vi "DisplayCurrentValues.vi"(8 "error in (no error)":errorcluster, 11 "Tare Currents?":bool) -> (0 "error out":errorcluster, 1 "PDP Energy (J)":dbl, 2 "PDP Current (A)":dbl[](array[numeric]), 3 "Sum of Current":dbl, 4 "PDP Power (W)":dbl)   [LabVIEW 2016]
panel:
  in  "Reset Energy?":bool
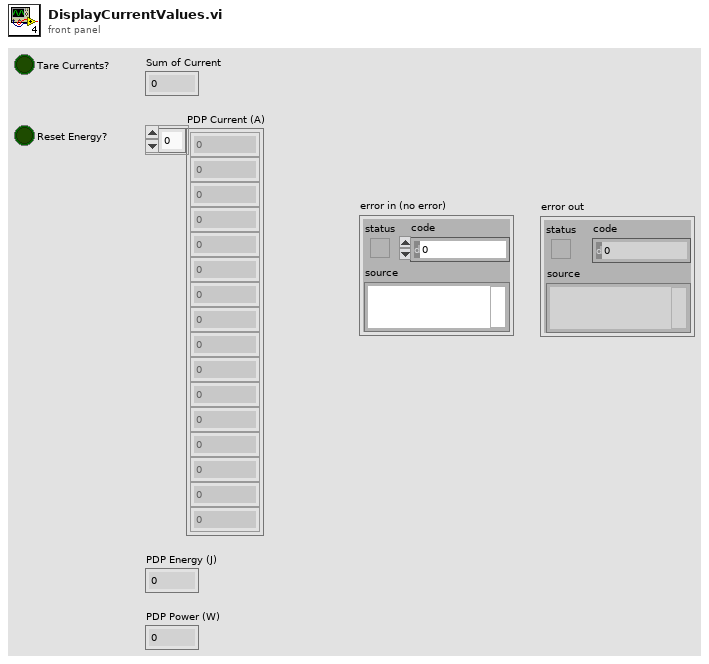
[diagram p1: front panel]
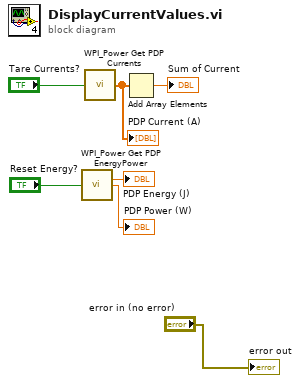
[diagram p0: block diagram]
diagram:
  n1 = call <vilib>:"WPI_Power Get PDP EnergyPower.vi"("Reset Energy?"="Reset Energy?") -> ("Energy (J)"=→"PDP Energy (J)":dbl, "Power (W)"=→"PDP Power (W)":dbl)  [unwired: 12 in, 1 out]
  n2 = call <vilib>:"WPI_Power Get PDP Currents.vi"("Tare Currents?"="Tare Currents?") -> ("all currents (A)"=w4:dbl[])  [unwired: 12 in, 2 out]
  "PDP Current (A)" <- w4
  n3 = Add Array Elements(numeric array=w4) -> (sum=→"Sum of Current":dbl)
  "error out" <- "error in (no error)"
